vi "ConnectionHelper.vi"(8 "ErrorIn":errorcluster, 9 "Disconnect":bool, 10 "Setting":u32, 11 "InCluster":T2) -> (0 "ErrorOut":errorcluster, 1 "Disconnected":bool, 3 "OutCluster":T1)   [LabVIEW 2022 SP3]
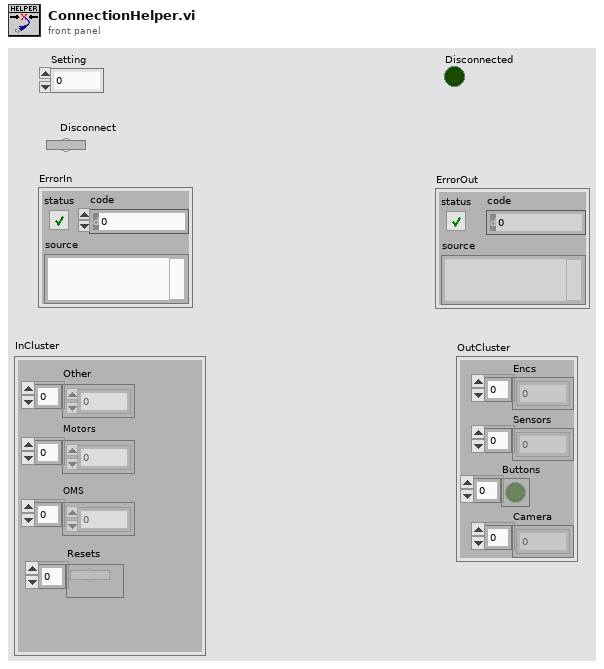
[diagram p1: front panel]
types:
  T1 = cluster{"Encs":dbl[], "Sensors":dbl[], "Buttons":bool[], "Camera":u8[]}
  T2 = cluster{"Other":dbl[], "Motors":dbl[], "OMS":dbl[], "Resets":bool[]}
  T3 = cluster{"Array":dbl[], "Array":dbl[], "Array":bool[], "OutBytes":u8[]}
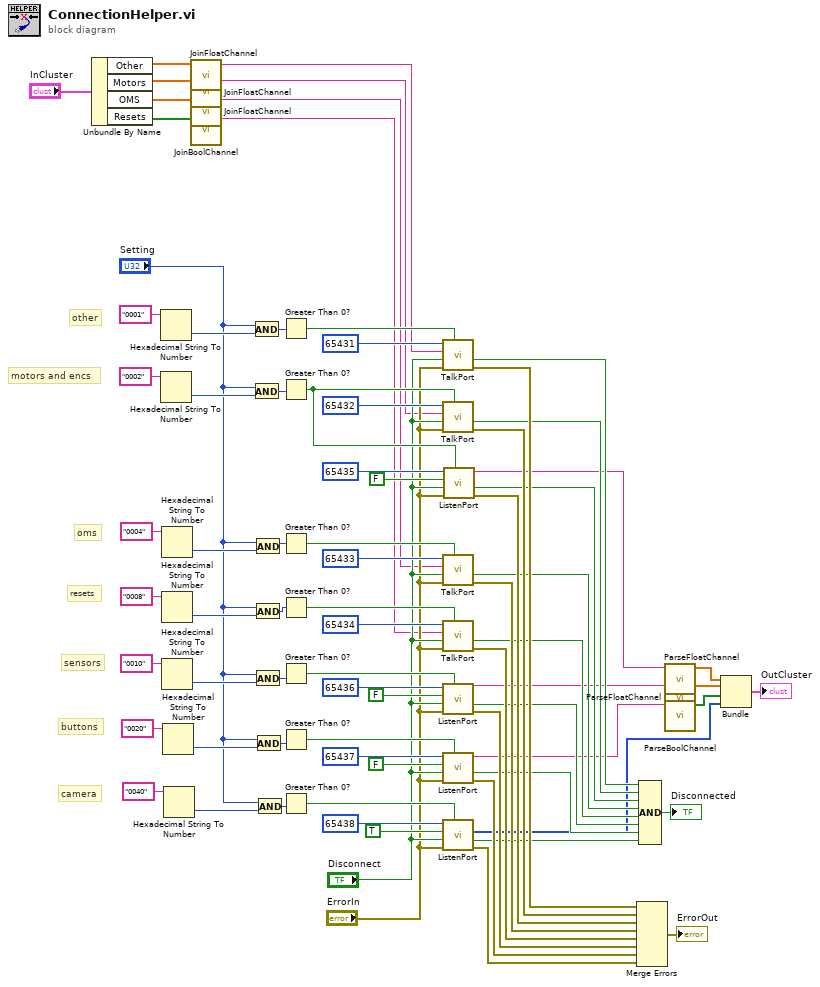
[diagram p0: block diagram]
diagram:
  # "camera"
  # "buttons"
  # "sensors"
  # "resets"
  # "oms"
  # "motors and encs"
  # "other"
  n1 = Unbundle By Name("InCluster") -> ("Other"=w14:dbl[], "Motors"=w12:dbl[], "OMS"=w10:dbl[], "Resets"=w8:bool[])
  n2 = Hexadecimal String To Number(string="0001") -> (number=w78:u32)  [unwired: 2 in, 1 out]
  n3 = Hexadecimal String To Number(string="0002") -> (number=w75:u32)  [unwired: 2 in, 1 out]
  n4 = Hexadecimal String To Number(string="0004") -> (number=w74:u32)  [unwired: 2 in, 1 out]
  n5 = Hexadecimal String To Number(string="0008") -> (number=w72:u32)  [unwired: 2 in, 1 out]
  n6 = Hexadecimal String To Number(string="0010") -> (number=w70:u32)  [unwired: 2 in, 1 out]
  n7 = Hexadecimal String To Number(string="0020") -> (number=w68:u32)  [unwired: 2 in, 1 out]
  n8 = Hexadecimal String To Number(string="0040") -> (number=w66:u32)  [unwired: 2 in, 1 out]
  n9 = call "JoinFloatChannel.vi"("Array"=w14) -> ("String"=w15:string)  [unwired: 10 in]
  n10 = call "JoinFloatChannel.vi"("Array"=w12) -> ("String"=w13:string)  [unwired: 10 in]
  n11 = call "JoinFloatChannel.vi"("Array"=w10) -> ("String"=w11:string)  [unwired: 10 in]
  n12 = call "JoinBoolChannel.vi"("Array"=w8) -> ("String"=w9:string)  [unwired: 10 in]
  n13 = And(x="Setting", y=w78) -> (x .and. y?=w63:u32)
  n14 = And(x="Setting", y=w75) -> (x .and. y?=w62:u32)
  n15 = And(x="Setting", y=w74) -> (x .and. y?=w61:u32)
  n16 = And(x="Setting", y=w72) -> (x .and. y?=w60:u32)
  n17 = And(x="Setting", y=w70) -> (x .and. y?=w59:u32)
  n18 = And(x="Setting", y=w68) -> (x .and. y?=w58:u32)
  n19 = And(x="Setting", y=w66) -> (x .and. y?=w57:u32)
  n20 = Greater Than 0?(x=w63) -> (x > 0?=w56:bool)
  n21 = Greater Than 0?(x=w62) -> (x > 0?=w50:bool)
  n22 = Greater Than 0?(x=w61) -> (x > 0?=w55:bool)
  n23 = Greater Than 0?(x=w60) -> (x > 0?=w54:bool)
  n24 = Greater Than 0?(x=w59) -> (x > 0?=w53:bool)
  n25 = Greater Than 0?(x=w58) -> (x > 0?=w52:bool)
  n26 = Greater Than 0?(x=w57) -> (x > 0?=w51:bool)
  n27 = call "TalkPort.vi"("IsEnabled"=w56, "error constant"="ErrorIn", "StopThread"="Disconnect", "OutString"=w15, "Port"=u16 65431) -> ("error out"=w35:errorcluster, "Socket Closed"=w26:bool)  [unwired: 4 in]
  n28 = call "TalkPort.vi"("IsEnabled"=w50, "error constant"="ErrorIn", "StopThread"="Disconnect", "OutString"=w13, "Port"=u16 65432) -> ("error out"=w34:errorcluster, "Socket Closed"=w25:bool)  [unwired: 4 in]
  n29 = call "TalkPort.vi"("IsEnabled"=w55, "error constant"="ErrorIn", "StopThread"="Disconnect", "OutString"=w11, "Port"=u16 65433) -> ("error out"=w32:errorcluster, "Socket Closed"=w23:bool)  [unwired: 4 in]
  n30 = call "TalkPort.vi"("IsEnabled"=w54, "error constant"="ErrorIn", "StopThread"="Disconnect", "OutString"=w9, "Port"=u16 65434) -> ("error out"=w31:errorcluster, "Socket Closed"=w22:bool)  [unwired: 4 in]
  n31 = call "ListenPort.vi"("IsEnabled"=w53, "error constant"="ErrorIn", "StopThread"="Disconnect", "IsCamera"=FALSE, "Port"=u16 65436) -> ("error out"=w30:errorcluster, "Socket Closed"=w21:bool, "OutString"=w4:string)  [unwired: 3 in, 1 out]
  n32 = call "ListenPort.vi"("IsEnabled"=w52, "error constant"="ErrorIn", "StopThread"="Disconnect", "IsCamera"=FALSE, "Port"=u16 65437) -> ("error out"=w29:errorcluster, "Socket Closed"=w20:bool, "OutString"=w2:string)  [unwired: 3 in, 1 out]
  n33 = call "ListenPort.vi"("IsEnabled"=w51, "error constant"="ErrorIn", "StopThread"="Disconnect", "IsCamera"=TRUE, "Port"=u16 65438) -> ("error out"=w28:errorcluster, "Socket Closed"=w19:bool, "OutBytes"=w16:u8[])  [unwired: 3 in, 1 out]
  n34 = call "ListenPort.vi"("IsEnabled"=w50, "error constant"="ErrorIn", "StopThread"="Disconnect", "IsCamera"=FALSE, "Port"=u16 65435) -> ("error out"=w33:errorcluster, "Socket Closed"=w24:bool, "OutString"=w6:string)  [unwired: 3 in, 1 out]
  n35 = Merge Errors(w35, w34, w33, w32, w31, w30, w29, w28) -> (→"ErrorOut":errorcluster)
  n36 = Compound Arithmetic op=AND(w26, w25, w24, w23, w22, w21, w20, w19) -> (→"Disconnected":bool)
  n37 = call "ParseFloatChannel.vi"("Input"=w6) -> ("Array"=w7:dbl[])  [unwired: 10 in]
  n38 = call "ParseFloatChannel.vi"("Input"=w4) -> ("Array"=w5:dbl[])  [unwired: 10 in]
  n39 = call "ParseBoolChannel.vi"("Input"=w2) -> ("Array"=w3:bool[])  [unwired: 10 in]
  n40 = Bundle("Array"=w7, "Array"=w5, "Array"=w3, "OutBytes"=w16) -> (→"OutCluster":T3)  [unwired: 1 in]
